vi "Populate Baudrates.vi"(8 "error in":errorcluster, 11 "UI Actor in":refnum<class "UI Actor.lvclass">) -> (0 "error out":errorcluster)   [LabVIEW 2019, in "UI Actor.lvlib" / "UI Actor.lvclass"]
uses:
  UI Actor.lvclass
  UI Actor.lvclass/UI Actor.ctl
  Controls/Supported Baudrates.ctl
  UI Actor.lvlib
  Electronic Datasheet/Electronic Datasheet.lvclass
  Core/Device Info/Device Info.lvclass
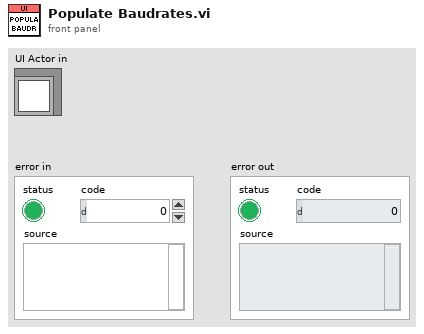
[diagram p1: front panel]
types:
  T1 = typedef "UI Actor.lvlib/Supported Baudrates.ctl" = cluster{"BaudRate_10":bool, "BaudRate_20":bool, "BaudRate_50":bool, "BaudRate_125":bool, "BaudRate_250":bool, "BaudRate_500":bool, "BaudRate_800":bool, "BaudRate_1000":bool, "BaudRate_auto":bool}
  T2 = map{path, refnum<class "Electronic Datasheet.lvclass">}
  T3 = cluster{"VendorName":string, "VendorNumber":u32, "ProductName":string, "ProductNumber":u32, "RevisionNumber":u32, "OrderCode":string, "BaudRate_10":bool, "BaudRate_20":bool, "BaudRate_50":bool, "BaudRate_125":bool, "BaudRate_250":bool, "BaudRate_500":bool, "BaudRate_800":bool, "BaudRate_1000":bool, "BaudRate_auto":bool, "SimpleBootUpMaster":bool, "SimpleBootUpSlave":bool, "Granularity":u8, "DynamicChannelsSupported":bool, "CompactPDO":u8, "GroupMessaging":bool, "NrOfRXPDO":u16, "NrOfTXPDO":u16, "LSS_Supported":bool, "LSS_Master":bool, "NG_Slave":bool, "NG_Master":bool, "NrOfNG_MonitoredNodes":u16}
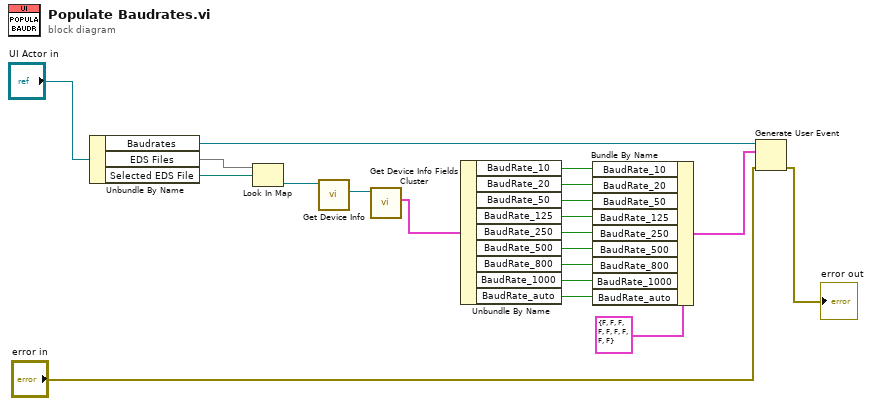
[diagram p0: block diagram]
diagram:
  n1 = Unbundle By Name("UI Actor in") -> ("Baudrates"=w20:refnum<user-event>, "EDS Files"=w17:T2, "Selected EDS File"=w15:path)
  n2 = Look In Map(map=w17, key=w15) -> (value=w16:refnum<class "Electronic Datasheet.lvclass">)  [unwired: 1 in, 1 out]
  n3 = call "Get Device Info.vi"("reference in"=w16) -> ("Device Info"=w14:refnum<class "Device Info.lvclass">)  [unwired: 8 in, 2 out]
  n4 = call "Get Device Info Fields Cluster.vi"("Device Info in"=w14) -> ("Device Info"=w12:T3)  [unwired: 9 in, 1 out]
  n5 = Unbundle By Name(w12) -> ("BaudRate_10"=w9:bool, "BaudRate_20"=w8:bool, "BaudRate_50"=w7:bool, "BaudRate_125"=w6:bool, "BaudRate_250"=w5:bool, "BaudRate_500"=w4:bool, "BaudRate_800"=w3:bool, "BaudRate_1000"=w2:bool, "BaudRate_auto"=w1:bool)
  n6 = Bundle By Name(cluster=T1 {"BaudRate_10"=FALSE, "BaudRate_20"=FALSE, "BaudRate_50"=FALSE, "BaudRate_125"=FALSE, "BaudRate_250"=FALSE, "BaudRate_500"=FALSE, "BaudRate_800"=FALSE, "BaudRate_1000"=FALSE, "BaudRate_auto"=FALSE} ("Baudrates"), "BaudRate_10"=w9, "BaudRate_20"=w8, "BaudRate_50"=w7, "BaudRate_125"=w6, "BaudRate_250"=w5, "BaudRate_500"=w4, "BaudRate_800"=w3, "BaudRate_1000"=w2, "BaudRate_auto"=w1) -> (w10:T1)
  n7 = Generate User Event(user event=w20, event data cluster=w10, error in="error in") -> (error out=→"error out":errorcluster)  [unwired: 1 in, 1 out]
